vi "oa_SCL Plot XY.vi"(0 "picture":picture, 1 "desired font(Application)":T5(ring)=enum."Application Font", 3 "[user-specified font]":T6, 5 "data":cluster{"x":dbl, "y":dbl}[](array[cluster]) {"y" format="%0.2f"; "x" format="%0.2f"}, 7 "dimensions (w,h)":cluster{"width":i16, "height":i16}, 11 "top left point(0, 0)":cluster{"x":i16, "y":i16}, 12 "cartesian axis attributes":T7={"x minimum"=0.0, "x maximum"=0.0, "x log?"=FALSE, "x precision"=1, "x format"=enum."Decimal", "y minimum"=0.0, "y maximum"=0.0, "y log?"=FALSE, "y precision"=1, "y format"=enum."Decimal"} {"x minimum" format="%0.2f"; "x maximum" format="%0.2f"; "y minimum" format="%0.2f"; "y maximum" format="%0.2f"}, 13 "cartesian grid cosmetics":T4={"line color"=6710886, "text color"=13421772, "tick length(3)"=3, "crossing axes"=FALSE, "visible grid?"=TRUE}, 14 "XY plot cosmetics":T3={"plot color"=16776960, "XY plot type"=enum."connected points", "baseline"=0.0} {"baseline" format="%0.2f"}, 15 "[sized scatter plot cosmetics]":T1={"min size"=1, "max size"=5, "maps to max size"=5, "color array"=[16776960, 65280, 16711680, 255]}) -> (4 "new picture":picture, 6 "x scale factors":cluster{"a":dbl, "b":dbl, "log?":bool} {"b" format="%0.2f"; "a" format="%0.2f"}, 8 "y scale factors":cluster{"a":dbl, "b":dbl, "log?":bool} {"b" format="%0.2f"; "a" format="%0.2f"})   [LabVIEW 2017]
uses:
  <vilib>/picture/cartesn2.llb/XY Plot Type.ctl
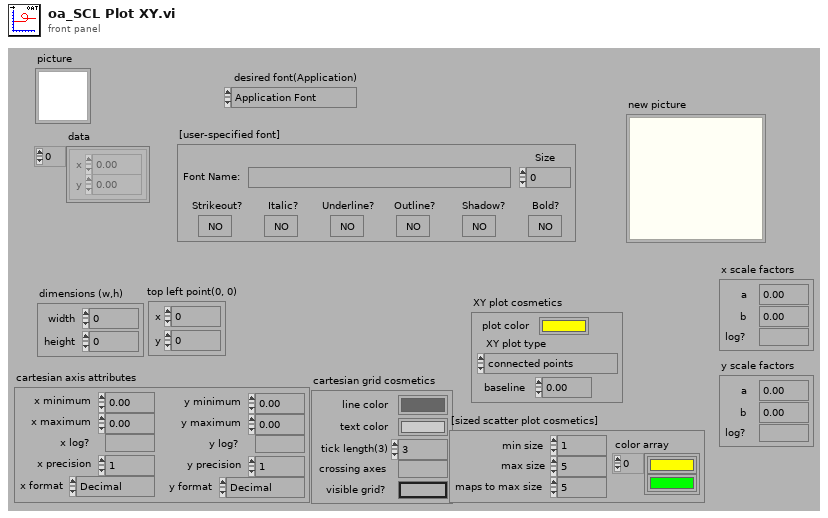
[diagram p1: front panel]
types:
  T1 = cluster{"min size":i16, "max size":i16, "maps to max size":i16, "color array":u32[]}
  T2 = typedef "XY Plot Type.ctl" = enum16{"points", "squares", "circles", "connected points", "connected squares", "connected circles", "comb plot", "sized scatter plot", "sized-colored scatter plot", "min-max lines"}
  T3 = cluster{"plot color":u32, "XY plot type":T2, "baseline":dbl}
  T4 = cluster{"line color":u32, "text color":u32, "tick length(3)":i16, "crossing axes":bool, "visible grid?":bool}
  T5 = enum16{"User-specified Font", "Application Font", "System Font", "Dialog Font"}
  T6 = cluster{"Font Name:":string, "Size":i16, "Strikeout?":bool, "Italic?":bool, "Underline?":bool, "Outline?":bool, "Shadow?":bool, "Bold?":bool}
  T7 = cluster{"x minimum":dbl, "x maximum":dbl, "x log?":bool, "x precision":u8, "x format":enum8{"Decimal", "Scientific", "Engineering", "Binary", "Octal", "Hex"}, "y minimum":dbl, "y maximum":dbl, "y log?":bool, "y precision":u8, "y format":enum8{"Decimal", "Scientific", "Engineering", "Binary", "Octal", "Hex"}}
  T8 = cluster{"left":i16, "top":i16, "right":i16, "bottom":i16}
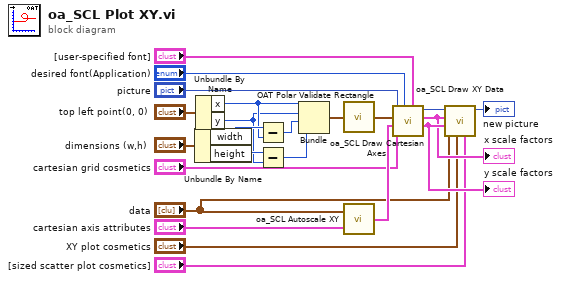
[diagram p0: block diagram]
diagram:
  n1 = Unbundle By Name("dimensions (w,h)") -> ("width"=w6:i16, "height"=w3:i16)
  n2 = Unbundle By Name("top left point(0, 0)") -> ("x"=w5:i16, "y"=w2:i16)
  n3 = Subtract(x=w6, y=w5) -> (x-y=w4:i16)
  n4 = Subtract(x=w3, y=w2) -> (x-y=w1:i16)
  n5 = Bundle("x"=w5, "y"=w2, w4, w1) -> (w9:cluster{"x":i16, "y":i16, i16, i16})  [unwired: 1 in]
  n6 = call <vilib>:"OAT Polar Validate Rectangle.vi"("rect"=w9) -> ("valid rect"=w21:T8)
  n7 = call <vilib>:"oa_SCL Autoscale XY.vi"("axis attributes"="cartesian axis attributes", "xy data"="data") -> ("axis attributes"=w22:T7)
  n8 = call <vilib>:"oa_SCL Draw Cartesian Axes.vi"("[user-specified font]"="[user-specified font]", "desired font(Application)"="desired font(Application)", "grid cosmetics"="cartesian grid cosmetics", "axis attributes"=w22, "bounding rect"=w21, "picture"="picture") -> ("y scale factors"=w17:cluster{"a":dbl, "b":dbl, "log?":bool}, "x scale factors"=w16:cluster{"a":dbl, "b":dbl, "log?":bool}, "new picture"=w14:picture)  [unwired: 3 in]
  "x scale factors" <- w16
  "y scale factors" <- w17
  n9 = call <vilib>:"oa_SCL Draw XY Data.vi"("[sized scatter plot cosmetics]"="[sized scatter plot cosmetics]", "xy cosmetics"="XY plot cosmetics", "xy data"="data", "y scale factors"=w17, "x scale factors"=w16, "picture"=w14) -> ("new picture"=→"new picture":picture)  [unwired: 5 in]
